vi "DISP_WIND_TRAC_TITL_DATA.vi"(0 "VISA IN":refnum<visa-resource-name>, 1 "Trace":i32=1, 2 "Title":string, 5 "error in":errorcluster, 7 "Window":i32=1) -> (14 "VISA Out":refnum<visa-resource-name>, 19 "error out":errorcluster)   [LabVIEW 2018, in "PNA-X.lvlib"]
doc: "DISPlay:WINDow<wnum>:TRACe<tnum>TITLe:DATA <string> \n1597\n\n(Read-Write) Writes and read data to the trace title area. The trace title is embedded in the trace status \nfield. Learn more. \nNewer entries replace (not append) older entries. The title is turned ON and OFF with \nDISP:WIND:TRAC:TITL:STAT. \nParameters \n<wnum> Any existing window number. If unspecified, value is set to 1. \n<tnum> Trace number of the specified window. If unspecified, value is set to 1. The \ntrace number displayed in trace status is the trace number of the channel; not \nthe window. Use Display:Cat? to read the window numbers. Use \nDisp:Window:Cat? to read the trace numbers of the specified window. \n<string> Title to be displayed. Any characters (not spaces) enclosed with quotes. \nExamples DISP:WIND:TRAC:TITL:DATA 'MyNewMeas' \ndisplay:window2:trace3:title:data 'hello' \nQuery Syntax DISPlay:WINDow<wnum>:TRACe<tnum>TITLe:DATA? \nReturn Type String \nDefault Not Applicable"
uses:
  PNA-X.lvlib
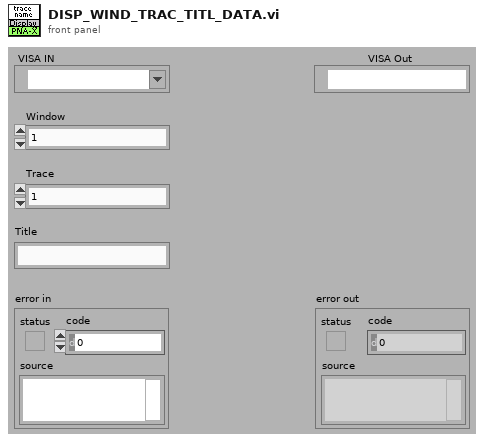
[diagram p1: front panel]
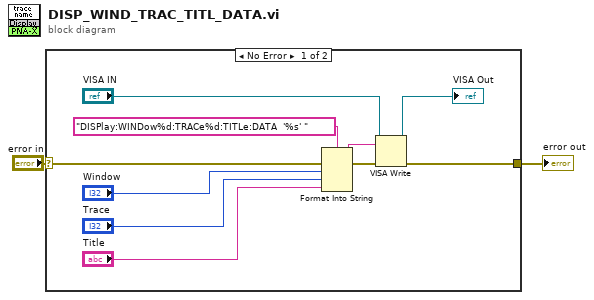
[diagram p0: block diagram]
diagram:
  n1 = case shown="No Error" "error in" {
    selector: "error in" -> [w12 w13]
    tunnel: [w7 w13] -> w1
    frame No Error {
      n2 = Format Into String(format string="DISPlay:WINDow%d:TRACe%d:TITLe:DATA  '%s' " ("Cmdline"), error in=w12, "Window", "Trace", "Title") -> (resulting string=w10:string, error out=w11:errorcluster)  [unwired: 1 in]
      n3 = VISA Write(VISA resource name="VISA IN", write buffer=w10, error in (no error)=w11) -> (VISA resource name out=→"VISA Out":refnum<visa-resource-name>, error out=w7:errorcluster)  [unwired: 1 out]
    }
    frame Error {
    }
  }
  "error out" <- w1
